vi "Levelmeter_shield_vergleich.vi"(4 "Shield Level (%)":i32=50 max=100 step=10, 5 "Automatic Shield refill activatet":bool, 6 "LN Shield Refill activatet":bool) -> (1 "Data out":bool)   [LabVIEW 2019]
uses:
  Global/Global Variables/Data_Display_global.vi
  Instrument_Setup.vi
panel:
  out "wait for n_shield [min]":dbl
  out "max filltime n_shield [min]":dbl=25.0
  out "max_n_shield":i32=100 min=0 max=100 step=10
  out "min_n_shield":i32=50 min=0 max=100 step=10
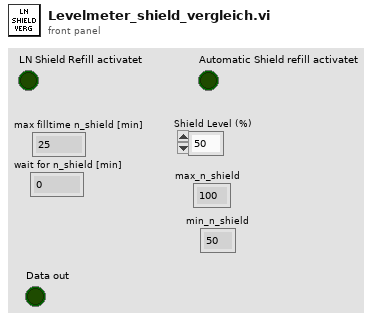
[diagram p1: front panel]
types:
  T1 = cluster{"max filltime Shield (min)":dbl, "wait for Shield (min)":dbl, "min Shield (%)":dbl, "max Shield (%)":dbl, "max filltime Trap":dbl, "min Coldtrap (%)":dbl, "wait for Coldtrap (min)":dbl, "max Coldtrap (%)":dbl}
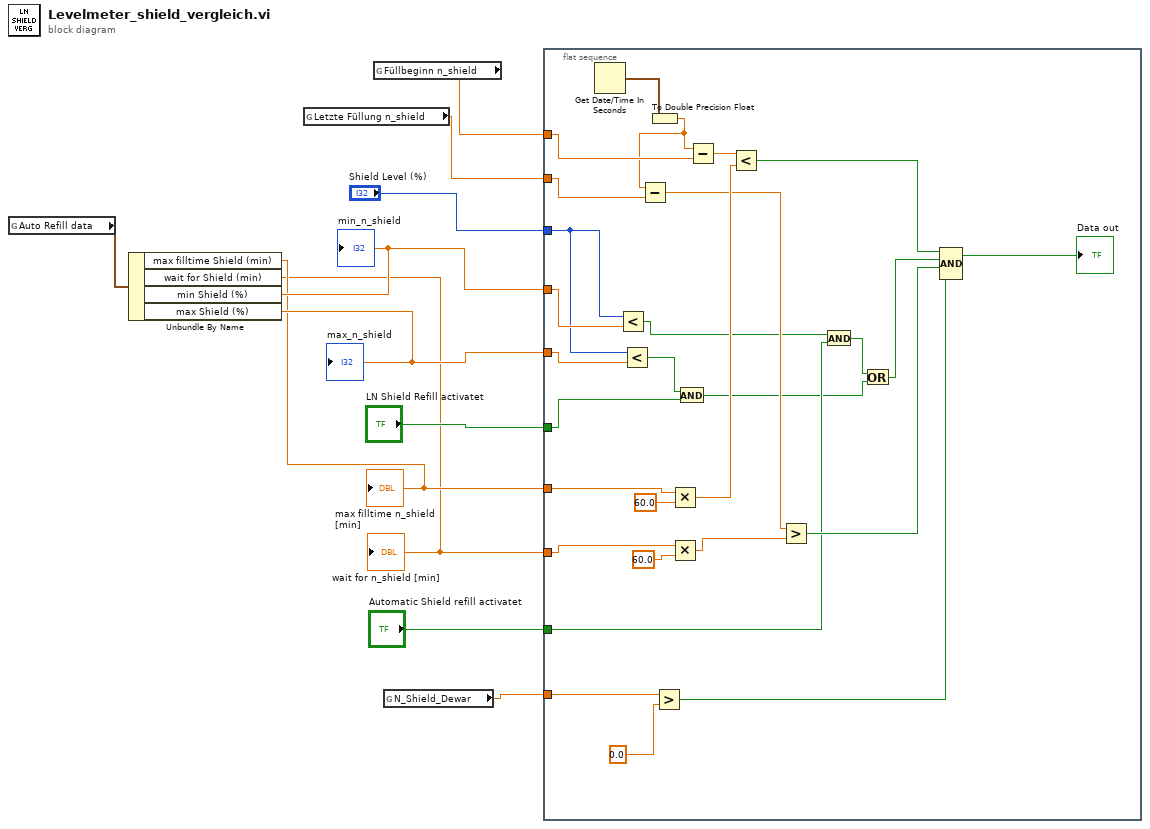
[diagram p0: block diagram]
diagram:
  n1 = global read "Instrument_Setup.vi" "Auto Refill data"() -> (w6:T1)
  n2 = Unbundle By Name(w6) -> ("max filltime Shield (min)"=w3:dbl, "wait for Shield (min)"=w2:dbl, "min Shield (%)"=w5:dbl, "max Shield (%)"=w4:dbl)
  "min_n_shield" <- w5
  "max_n_shield" <- w4
  "max filltime n_shield [min]" <- w3
  "wait for n_shield [min]" <- w2
  n3 = global read "Data_Display_global.vi" "Letzte Füllung n_shield"() -> (w10:dbl)
  n4 = global read "Data_Display_global.vi" "Füllbeginn n_shield"() -> (w11:dbl)
  n5 = global read "Data_Display_global.vi" "N_Shield_Dewar"() -> (w1:dbl)
  n6 = flat-sequence {
    tunnel: w11 -> [w38]
    tunnel: w10 -> [w30]
    tunnel: "Shield Level (%)" -> [w23]
    tunnel: w5 -> [w25]
    tunnel: w4 -> [w24]
    tunnel: "LN Shield Refill activatet" -> [w21]
    tunnel: w3 -> [w35]
    tunnel: w2 -> [w32]
    tunnel: "Automatic Shield refill activatet" -> [w19]
    tunnel: w1 -> [w14]
    frame #0 {
      n7 = Get Date/Time In Seconds() -> (seconds since 1Jan1904=w39:timestamp)
      n8 = Less?(x=w23, y=w25) -> (x < y?=w20:bool)
      n9 = Less?(x=w23, y=w24) -> (x < y?=w22:bool)
      n10 = To Double Precision Float(number=w39) -> (double precision float=w29:dbl)
      n11 = Subtract(x=w29, y=w30) -> (x-y=w28:dbl)
      n12 = Greater?(x=w14, y=0.0) -> (0:w12:bool)
      n13 = Multiply(x=w35, y=60.0) -> (x*y=w34:dbl)
      n14 = Multiply(x=w32, y=60.0) -> (x*y=w31:dbl)
      n15 = And(x=w22, y=w21) -> (x .and. y?=w17:bool)
      n16 = Subtract(x=w29, y=w38) -> (x-y=w37:dbl)
      n17 = Less?(x=w37, y=w34) -> (x < y?=w27:bool)
      n18 = Greater?(x=w28, y=w31) -> (0:w26:bool)
      n19 = And(x=w20, y=w19) -> (x .and. y?=w18:bool)
      n20 = Or(x=w18, y=w17) -> (x .or. y?=w16:bool)
      n21 = Compound Arithmetic op=AND ("Mehrfacharithmetik")(w27, w16, w26, w12) -> (→"Data out":bool)
    }
  }
